vi "1002246 Telit play with rts cts.vi"(8 "error in (no error)":errorcluster) -> (0 "error out":errorcluster, 1 "RTS control ok?":bool, 3 "PassFail":string, 4 "Comport responsive?":bool, 5 "Comport unresponsive?":bool)   [LabVIEW 2013]
uses:
  NanoArduino/NanoCmds.ctl
  Test Globals/Global 1.vi
panel:
  out "read buffer":string
  out "VISA resource name out":refnum<visa-resource-name>
  out "read buffer 3":string
  out "read buffer 2":string
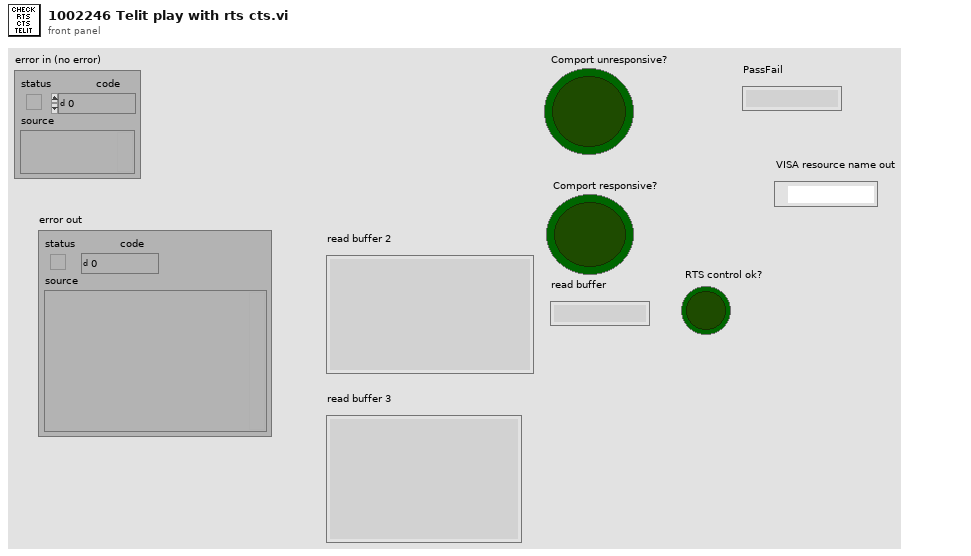
[diagram p1: front panel]
types:
  T1 = typedef "NanoCmds.ctl" = enum16{"Make digital port an output", "Make digital port an input", "Set digital pin high", "Set digital pin low", "Get digital pin state", "Get analog pin voltage", "Get analog pins difference", "Get ohms at analog pin", "Turn on current limit", "Reset Nano device", "Get digital pin state pullup", "Read current", "Initialize", "Power up uut", "Power down uut", "Get uut current draw", "Set ADC volts high", "Set ADC volts low", "Start up uut modem", "Get CTS state", "Get on_nsleep state", "Reset modem", "Get lid state", "Wait for lid closed", "Wait for lid open", "Power up, start, get curr", "Check if X2 shorted", "Power up and start up", "Check X3 shorted", "Get RTS state", "Get DTR state", "Reboot 1002759"}
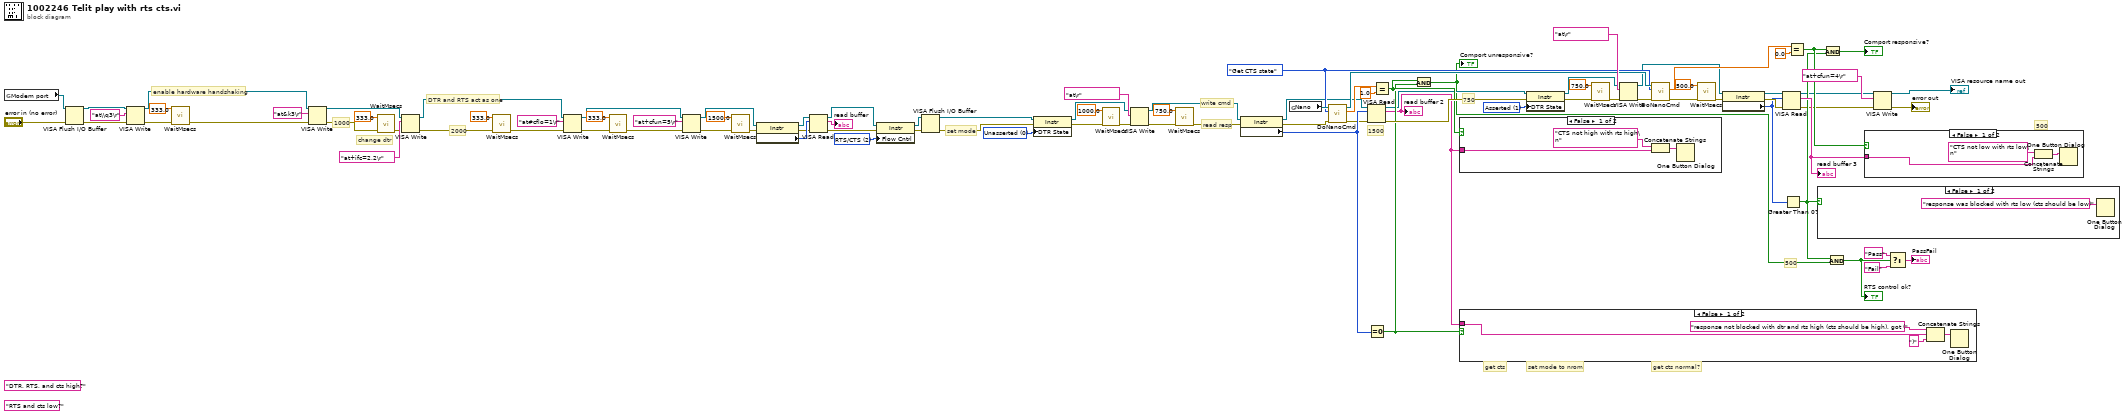
[diagram p0: block diagram]
diagram:
  (unwired) "RTS and cts low?" ("Message")
  (unwired) "DTR, RTS, and cts high?" ("Message")
  w60 = u16 2 items=["None", "XON/XOFF", "RTS/CTS", "XON/XOFF & RTS/CTS", "DTR/DSR", "XON/XOFF & DTR/DSR"] ("Serial Settings:Flow Control")
  w66 = NanoCmds."Get CTS state" ("Nano Op")
  w89 = i16 1 items=["Unknown"=-1, "Unasserted"=0, "Asserted"=1] ("Serial Settings:Modem Line Settings:Line DTR State")
  w93 = i16 0 items=["Unknown"=-1, "Unasserted"=0, "Asserted"=1] ("Serial Settings:Modem Line Settings:Line DTR State")
  # "DTR and RTS act as one"
  # "500"
  # "500"
  # "750"
  # "1000"
  # "2000"
  # "1500"
  # "enable hardware handshaking"
  # "get cts normal?"
  # "set mode to nrom"
  # "read resp"
  # "get cts"
  # "write cmd"
  # "set mode"
  # "change dtr"
  n1 = global read "Global 1.vi" "Modem port"() -> (w54:refnum<visa-resource-name>)
  n2 = VISA Flush I/O Buffer(VISA resource name=w54, error in (no error)="error in (no error)") -> (VISA resource name out=w18:refnum<visa-resource-name>, error out=w17:errorcluster)  [unwired: 1 in]
  n3 = VISA Write(VISA resource name=w18, write buffer="at\\q3\r", error in (no error)=w17) -> (VISA resource name out=w13:refnum<visa-resource-name>, error out=w15:errorcluster)  [unwired: 1 out]
  n4 = call "WaitMsecs.vi"("error in (no error)"=w15, "Wait Msecs"=333.0) -> ("error out"=w14:errorcluster)  [unwired: 9 in]
  n5 = VISA Write(VISA resource name=w13, write buffer="at&k3\r", error in (no error)=w14) -> (VISA resource name out=w43:refnum<visa-resource-name>, error out=w33:errorcluster)  [unwired: 1 out]
  n6 = call "WaitMsecs.vi"("error in (no error)"=w33, "Wait Msecs"=333.0) -> ("error out"=w32:errorcluster)  [unwired: 9 in]
  n7 = VISA Write(VISA resource name=w43, write buffer="at+ifc=2,2\r", error in (no error)=w32) -> (VISA resource name out=w9:refnum<visa-resource-name>, error out=w11:errorcluster)  [unwired: 1 out]
  n8 = call "WaitMsecs.vi"("error in (no error)"=w11, "Wait Msecs"=333.0) -> ("error out"=w10:errorcluster)  [unwired: 9 in]
  n9 = VISA Write(VISA resource name=w9, write buffer="at#cflo=1\r", error in (no error)=w10) -> (VISA resource name out=w5:refnum<visa-resource-name>, error out=w2:errorcluster)  [unwired: 1 out]
  n10 = call "WaitMsecs.vi"("error in (no error)"=w2, "Wait Msecs"=333.0) -> ("error out"=w1:errorcluster)  [unwired: 9 in]
  n11 = VISA Write(VISA resource name=w5, write buffer="at+cfun=5\r", error in (no error)=w1) -> (VISA resource name out=w4:refnum<visa-resource-name>, error out=w6:errorcluster)  [unwired: 1 out]
  n12 = call "WaitMsecs.vi"("error in (no error)"=w6, "Wait Msecs"=1500.0) -> ("error out"=w37:errorcluster)  [unwired: 9 in]
  n13 = property class="Instr"(reference=w4, error in=w37) -> (reference out=w49:refnum<visa-resource-name>, error out=w48:errorcluster, "Serial Settings:Number of Bytes at Serial Port"=w50:u32)
  n14 = VISA Read(VISA resource name=w49, byte count=w50, error in (no error)=w48) -> (VISA resource name out=w40:refnum<visa-resource-name>, read buffer=→"read buffer":string, error out=w39:errorcluster)  [unwired: 1 out]
  n15 = property class="Instr"(reference=w40, error in=w39, "Flow Cntrl"=w60) -> (reference out=w53:refnum<visa-resource-name>, error out=w52:errorcluster)
  n16 = VISA Flush I/O Buffer(VISA resource name=w53, error in (no error)=w52) -> (VISA resource name out=w42:refnum<visa-resource-name>, error out=w41:errorcluster)  [unwired: 1 in]
  n17 = property class="Instr"(reference=w42, error in=w41, "DTR State"=w93) -> (reference out=w38:refnum<visa-resource-name>, error out=w35:errorcluster)
  n18 = call "WaitMsecs.vi"("error in (no error)"=w35, "Wait Msecs"=1000.0) -> ("error out"=w21:errorcluster)  [unwired: 9 in]
  n19 = VISA Write(VISA resource name=w38, write buffer="at\r", error in (no error)=w21) -> (VISA resource name out=w45:refnum<visa-resource-name>, error out=w59:errorcluster)  [unwired: 1 out]
  n20 = call "WaitMsecs.vi"("error in (no error)"=w59, "Wait Msecs"=750.0) -> ("error out"=w46:errorcluster)  [unwired: 9 in]
  n21 = property class="Instr"(reference=w45, error in=w46) -> (reference out=w65:refnum<visa-resource-name>, error out=w58:errorcluster, "Serial Settings:Number of Bytes at Serial Port"=w91:u32)
  n22 = global read "Global 1.vi" "Nano"() -> (w73:refnum<visa-resource-name>)
  n23 = call "DoNanoCmd.vi"("error in (no error)"=w58, "Nano Op"=w66, "VISA resource name"=w73) -> ("error out"=w57:errorcluster, "Read Value"=w72:dbl, "VISA resource name 2"=w70:refnum<visa-resource-name>)  [unwired: 5 in, 1 out]
  n24 = VISA Read(VISA resource name=w65, byte count=w91, error in (no error)=w57) -> (VISA resource name out=w64:refnum<visa-resource-name>, read buffer=w27:string, error out=w90:errorcluster)  [unwired: 1 out]
  "read buffer 2" <- w27
  n25 = Equal To 0?(x=w91) -> (x = 0?=w76:bool)
  n26 = Equal?(x=w72, y=1.0) -> (x = y?=w77:bool)
  n27 = And(x=w77, y=w76) -> (x .and. y?=w26:bool)
  "Comport unresponsive?" <- w26
  n28 = case shown="False" w77 {
    tunnel: w27 -> [w96 _]
    frame False {
      n29 = Concatenate Strings("CTS not high with rts high\n" ("message"), w96) -> (w95:string)
      n30 = One Button Dialog(message=w95) -> ()  [unwired: 1 in, 1 out]
    }
    frame True {
    }
  }
  n31 = case shown="False" w76 {
    tunnel: w27 -> [w100 _]
    frame False {
      n32 = Concatenate Strings("response not blocked with dtr and rts high (cts should be high), got (" ("message"), w100, ")" ("string")) -> (w98:string)
      n33 = One Button Dialog(message=w98) -> ()  [unwired: 1 in, 1 out]
    }
    frame True {
    }
  }
  n34 = property class="Instr"(reference=w64, error in=w90, "DTR State"=w89) -> (reference out=w63:refnum<visa-resource-name>, error out=w81:errorcluster)
  n35 = call "WaitMsecs.vi"("error in (no error)"=w81, "Wait Msecs"=750.0) -> ("error out"=w20:errorcluster)  [unwired: 9 in]
  n36 = VISA Write(VISA resource name=w63, write buffer="at\r", error in (no error)=w20) -> (VISA resource name out=w62:refnum<visa-resource-name>, error out=w69:errorcluster)  [unwired: 1 out]
  n37 = call "DoNanoCmd.vi"("error in (no error)"=w69, "Nano Op"=w66, "VISA resource name"=w70) -> ("error out"=w56:errorcluster, "Read Value"=w68:dbl)  [unwired: 5 in, 2 out]
  n38 = call "WaitMsecs.vi"("error in (no error)"=w56, "Wait Msecs"=500.0) -> ("error out"=w87:errorcluster)  [unwired: 9 in]
  n39 = property class="Instr"(reference=w62, error in=w87) -> (reference out=w61:refnum<visa-resource-name>, error out=w85:errorcluster, "Serial Settings:Number of Bytes at Serial Port"=w83:u32)
  n40 = VISA Read(VISA resource name=w61, byte count=w83, error in (no error)=w85) -> (VISA resource name out=w23:refnum<visa-resource-name>, read buffer=w44:string, error out=w22:errorcluster)  [unwired: 1 out]
  "read buffer 3" <- w44
  n41 = Greater Than 0?(x=w83) -> (x > 0?=w25:bool)
  n42 = Equal?(x=w68, y=0.0) -> (x = y?=w74:bool)
  n43 = case shown="False" w25 {
    frame False {
      n44 = One Button Dialog(message="response was blocked with rts low (cts should be low)") -> ()  [unwired: 1 in, 1 out]
    }
    frame True {
    }
  }
  n45 = And(x=w74, y=w25) -> (x .and. y?=→"Comport responsive?":bool)
  n46 = And(x=w25, y=w26) -> (x .and. y?=w24:bool)
  "RTS control ok?" <- w24
  n47 = case shown="False" w74 {
    tunnel: w44 -> [w104 _]
    frame False {
      n48 = Concatenate Strings("CTS not low with rts low\n" ("message"), w104) -> (w103:string)
      n49 = One Button Dialog(message=w103) -> ()  [unwired: 1 in, 1 out]
    }
    frame True {
    }
  }
  n50 = VISA Write(VISA resource name=w23, write buffer="at+cfun=4\r", error in (no error)=w22) -> (VISA resource name out=→"VISA resource name out":refnum<visa-resource-name>, error out=→"error out":errorcluster)  [unwired: 1 out]
  n51 = Select(t="Pass", s=w24, f="Fail") -> (s? t:f=→"PassFail":string)
